vi "Calculate Prescale.vi"(0 "minimum BER":dbl, 5 "in DFE mode?":bool, 7 "rx internal data width":T1=enum."32 Bit", 11 "error in":errorcluster) -> (4 "prescale":u8, 15 "error out":errorcluster)   [LabVIEW 2015, in "niHighSpeedSerial Eye Scan Common v1 Host.lvlib"]
doc: "Computes the prescale value given the specified <b>minimum BER</b> (Bit Error Rate) and Equalization Mode.\nBecause only discrete values are permitted for prescale, the calculated prescale value will likely result in a smaller Bit Error Rate than requested.\n\n<B>Input Parameters</B>\n\n<B>minimum BER</B> is the minimum bit error rate requested. Depending on the prescale calculation, the actual bit error rate is likely smaller.\n\n<B>in DFE mode?</B> is true if Eye Scan is configured for DFE Equalization Mode.\n\n<B>error in</B> describes error conditions that occur before this node runs. This input provides standard 'error in' functionality.\n\n<B>Output Parameters</B>\n\n<B>prescale</B> controls scaling of the sample count in order to keep the sample count and error count within reasonable precision.\n\n<B>error out</B> contains error information. This output provides standard 'error out' functionality."
uses:
  <instrlib>/niHighSpeedSerial/Eye Scan/v1/Host/Common/niHighSpeedSerial Eye Scan Common v1 Host.lvlib
  <instrlib>/niHighSpeedSerial/Eye Scan/v1/Host/Common/Public/Data Width.ctl
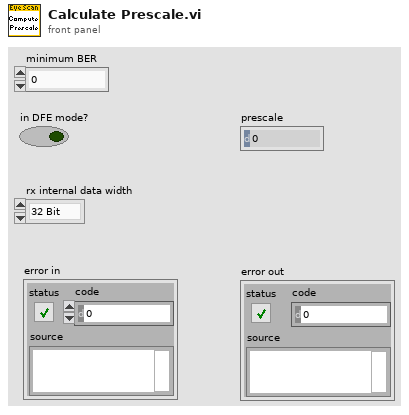
[diagram p1: front panel]
types:
  T1 = typedef "niHighSpeedSerial Eye Scan Common v1 Host.lvlib/Data Width.ctl" = enum16{"16 Bit", "20 Bit", "32 Bit", "40 Bit"}
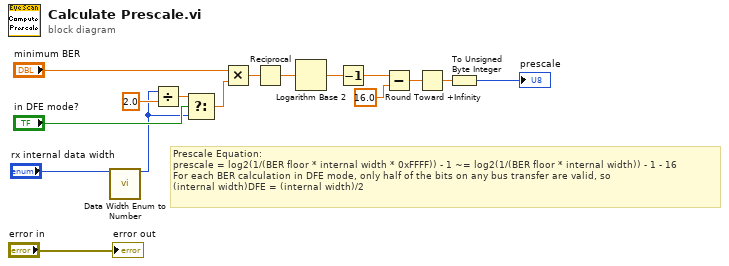
[diagram p0: block diagram]
diagram:
  # "Prescale Equation:\nprescale = log2(1/(BER floor * internal width * 0xFFFF)) - 1 ~= log2(1/(BER floor * internal width)) - 1 - 16\nFor each BER calculation in DFE mode, only half of the bits on any bus transfer are valid, so\n(internal width)DFE = (internal width)/2"
  n1 = call <instrlib>:"Data Width Enum to Number.vi"("receiver data width"="rx internal data width") -> ("numberic width"=w2:u64)  [unwired: 14 in]
  n2 = Divide(x=w2, y=2.0 ("x")) -> (x/y=w6:dbl)
  n3 = Select(t=w6, s="in DFE mode?", f=w2) -> (s? t:f=w5:dbl)
  n4 = Multiply(x="minimum BER", y=w5) -> (x*y=w7:dbl)
  n5 = Reciprocal(x=w7) -> (1/x=w14:dbl)
  n6 = Logarithm Base 2(1:w14) -> (0:w13:dbl)
  n7 = Decrement(x=w13) -> (x-1=w1:dbl)
  n8 = Subtract(x=w1, y=16.0 ("f")) -> (x-y=w11:dbl)
  n9 = Round Toward +Infinity(x=w11) -> (ceil(x): smallest int >= x=w9:dbl)
  n10 = To Unsigned Byte Integer(number=w9) -> (unsigned 8bit integer=→"prescale":u8)
  "error out" <- "error in"
